vi "Horizon.vi"(9 "Roll":dbl, 10 "Pitch":dbl, 11 "image data in":T1={"image type"=0, "image depth"=32, "image"=array[1123488 elements], "mask"=array[35856 elements], "colors"=[], "Rectangle"={"left"=0, "top"=0, "right"=282, "bottom"=996}}) -> (3 "2D Picture":picture)   [LabVIEW 2017, in "IL Driver Library.lvlib"]
uses:
  <vilib>/picture/picture.llb/imagedata.ctl
  IL Driver Library.lvlib
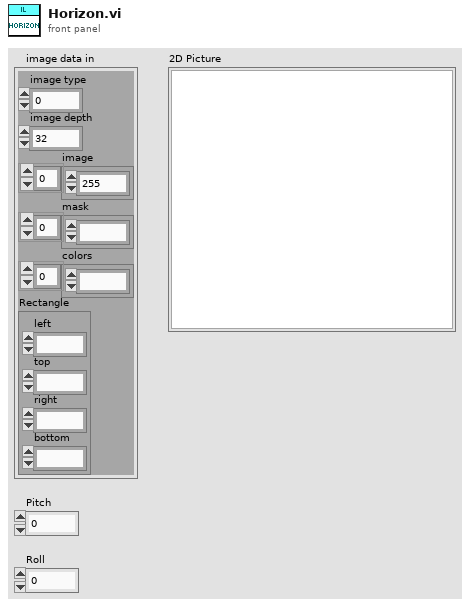
[diagram p1: front panel]
types:
  T1 = typedef "imagedata.ctl" = cluster{"image type":i32, "image depth":i32, "image":u8[], "mask":u8[], "colors":u32[], "Rectangle":cluster{"left":i16, "top":i16, "right":i16, "bottom":i16}}
  T2 = enum32{"Solid", "Dash", "Dot", "DashDot", "DashDotDot"}
  T3 = cluster{"вертикаль":i16, "Style":enum32{"Solid", "Dash", "Dot", "DashDot", "DashDotDot"}}
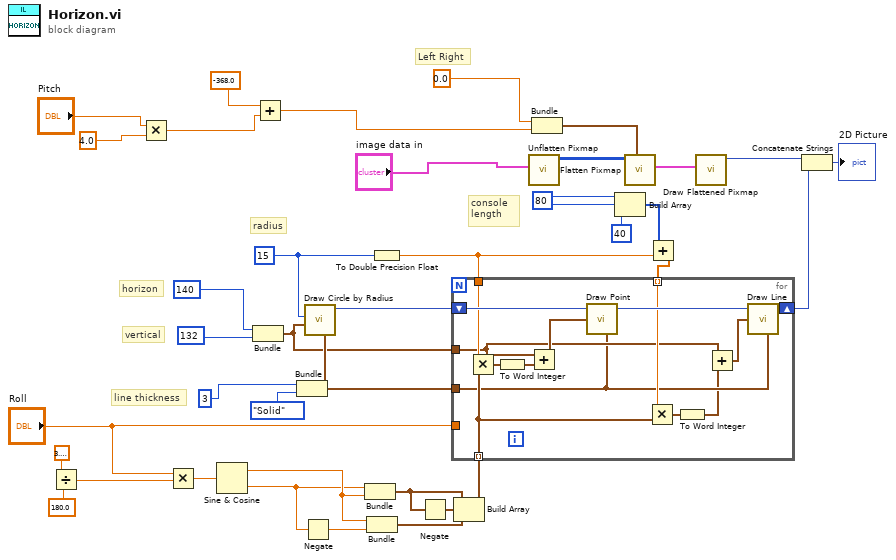
[diagram p0: block diagram]
diagram:
  w7 = i16 15 ("radius")
  w16 = i16 80 ("x")
  # "radius"
  # "line thickness"
  # "vertical"
  # "horizon"
  # "Left Right"
  # "console \nlength"
  n1 = Divide(x=3.141592653589793, y=180.0) -> (x/y=w35:dbl)
  n2 = Multiply(x="Pitch", y=4.0) -> (x*y=w3:dbl)
  n3 = Multiply(x="Roll", y=w35) -> (x*y=w20:dbl)
  n4 = Sine & Cosine(0:w20) -> (1:w13:dbl, 2:w12:dbl)
  n5 = Bundle("горизонталь"=i16 140, "вертикаль"=i16 132) -> (w10:cluster{"горизонталь":i16, "вертикаль":i16})  [unwired: 1 in]
  n6 = Add(x=-368.0, y=w3) -> (x+y=w5:dbl)
  n7 = Bundle("вертикаль"=i16 3, "Style"=T2."Solid") -> (w27:T3)  [unwired: 1 in]
  n8 = Negate(x=w12) -> (-x=w11:dbl)
  n9 = call <vilib>:"Draw Circle by Radius.vi"("pen"=w27, "pixel center"=w10, "radius"=w7) -> ("new picture"=w28:picture)  [unwired: 8 in]
  n10 = Bundle(w12, w13) -> (w19:cluster{dbl, dbl})  [unwired: 1 in]
  n11 = Bundle(w13, w11) -> (w17:cluster{dbl, dbl})  [unwired: 1 in]
  n12 = To Double Precision Float(number=w7) -> (double precision float=w6:dbl)
  n13 = Negate(x=w19) -> (-x=w18:cluster{dbl, dbl})
  n14 = Build Array(w19, w18, w17) -> (w14:cluster{dbl, dbl}[])
  n15 = call <vilib>:"Unflatten Pixmap.vi"("image data"="image data in") -> ("24-bit pixmap"=w33:u32[][])  [unwired: 4 in, 6 out]
  n16 = Bundle("x"=0.0, w5) -> (w32:cluster{"x":dbl, dbl})  [unwired: 1 in]
  n17 = Build Array(w16, w16, i16 40 ("x")) -> (w8:i16[])
  n18 = call <vilib>:"Flatten Pixmap.vi"("top left"=w32, "24-bit pixmap"=w33) -> ("image data"=w31:T1)  [unwired: 9 in]
  n19 = Add(x=w8, y=w6) -> (x+y=w9:dbl[])
  n20 = for {
    shift-right: [w50] -> w26
    shift-left: w28 -> [w51]
    tunnel: w27 -> [w41]
    tunnel: w14 -> [w45] mode=indexing
    tunnel: w9 -> [w46] mode=indexing
    tunnel: w6 -> [w49]
    tunnel: w10 -> [w44]
    tunnel: "Roll" -> [_]
    n21 = Multiply(x=w49, y=w45) -> (x*y=w48:cluster{dbl, dbl})
    n22 = To Word Integer(number=w48) -> (16bit integer=w40:cluster{i16, i16})
    n23 = Add(x=w44, y=w40) -> (x+y=w47:cluster{i16, i16})
    n24 = call <vilib>:"Draw Point.vi"("picture"=w51, "point(x,y)"=w47, "pen"=w41) -> ("new picture"=w52:picture)  [unwired: 6 in]
    n25 = Multiply(x=w46, y=w45) -> (x*y=w43:cluster{dbl, dbl})
    n26 = To Word Integer(number=w43) -> (16bit integer=w39:cluster{i16, i16})
    n27 = Add(x=w44, y=w39) -> (x+y=w42:cluster{i16, i16})
    n28 = call <vilib>:"Draw Line.vi"("picture"=w52, "end point"=w42, "pen"=w41) -> ("new picture"=w50:picture)  [unwired: 6 in]
  }
  n29 = call <vilib>:"Draw Flattened Pixmap.vi"("image data"=w31) -> ("new picture"=w30:picture)  [unwired: 8 in]
  n30 = Concatenate Strings(w30, w26) -> (→"2D Picture":picture)
